vi "ASCII to Unicode.vi"(9 "ASCII":string) -> (0 "interleaved array":u8[](array[numeric]), 1 "Unicode":string)   [LabVIEW 2015]
doc: "This code convert ASCII string characters to Unicode"
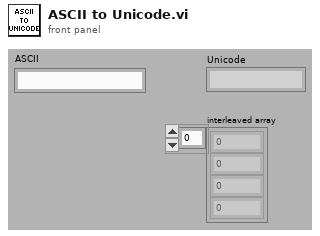
[diagram p1: front panel]
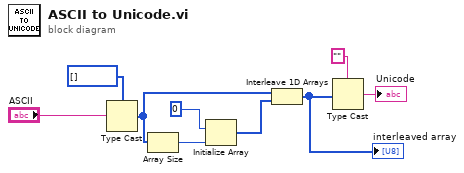
[diagram p0: block diagram]
diagram:
  n1 = Type Cast(type=u8[] [], x="ASCII") -> (*(type *) &x=w5:u8[])
  n2 = Array Size(array=w5) -> (size(s)=w7:i32)
  n3 = Initialize Array(u8 0, w7) -> (w4:u8[])
  n4 = Interleave 1D Arrays(w5, w4) -> (w3:u8[])
  "interleaved array" <- w3
  n5 = Type Cast(type="", x=w3) -> (*(type *) &x=→"Unicode":string)
